vi "Save File Create Default DOE Setup File.vi"(11 "Config Path":path=path "C:/GE/Washer DOE/WasherDOEConfig.csv") -> ()   [LabVIEW 2016, in "File Setup.lvlib"]
uses:
  File Setup.lvlib
  <vilib>/Utility/file.llb/Read From Spreadsheet File (string).vi
  <vilib>/Utility/file.llb/Write To Spreadsheet File (string).vi
panel:
  out "INI File Exists":bool
  out "CSV File Exists":bool
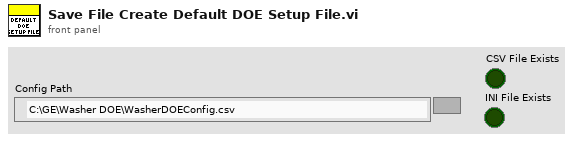
[diagram p1: front panel]
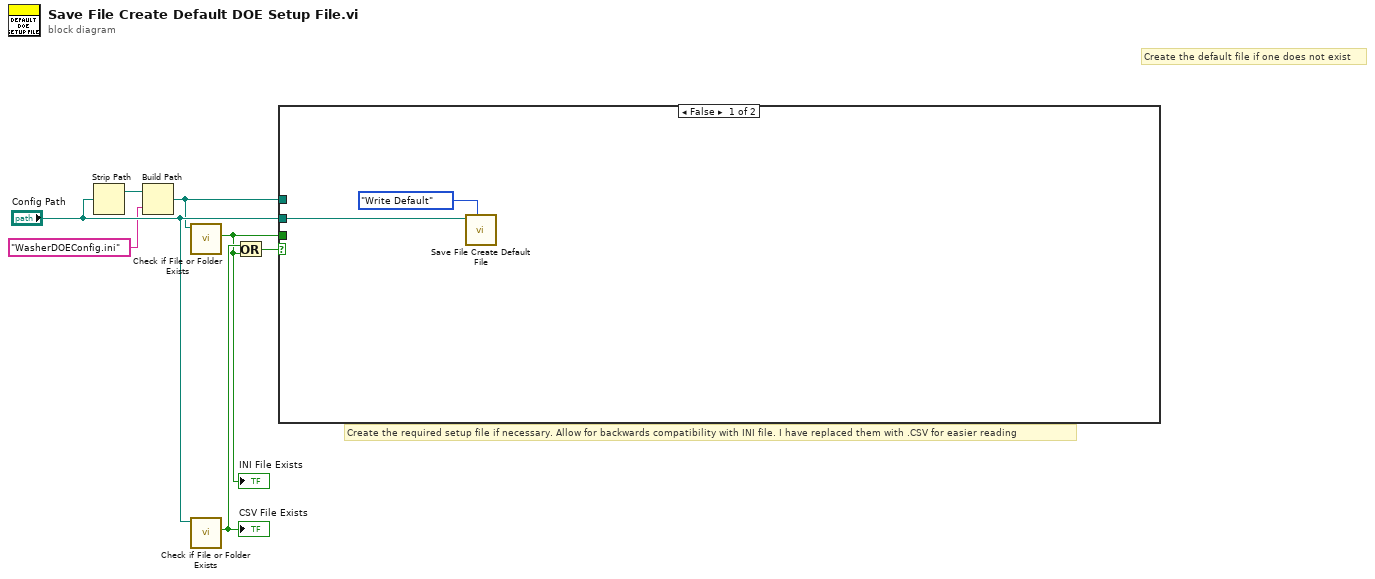
[diagram p0: block diagram]
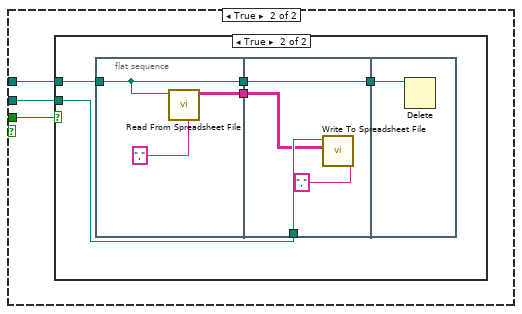
[diagram p2: hidden frame]
diagram:
  # "Create the required setup file if necessary. Allow for backwards compatibility with INI file. I have replaced them with .CSV for easier reading"
  # "Create the default file if one does not exist"
  n1 = Strip Path(path="Config Path") -> (stripped path=w4:path)  [unwired: 1 out]
  n2 = Build Path(base path=w4, name or relative path="WasherDOEConfig.ini") -> (appended path=w2:path)
  n3 = call <vilib>:"Check if File or Folder Exists.vi"("path"=w2) -> ("file or folder exists?"=w1:bool)  [unwired: 8 in, 2 out]
  "INI File Exists" <- w1
  n4 = call <vilib>:"Check if File or Folder Exists.vi"("path"="Config Path") -> ("file or folder exists?"=w7:bool)  [unwired: 8 in, 2 out]
  "CSV File Exists" <- w7
  n5 = Or(x=w7, y=w1) -> (x .or. y?=w6:bool)
  n6 = case shown="False" w6 {
    tunnel: "Config Path" -> [w9 w10]
    tunnel: w2 -> [_ w12]
    tunnel: w1 -> [_ w11]
    frame False {
      n7 = call "Save File Create Default File.vi"("Type"=enum16{"Pass Default", "Write Default"}."Write Default", "Config Path"=w9) -> ()  [unwired: 9 in, 1 out]
    }
    frame True {
      n8 = case shown="True" w11 {
        tunnel: w12 -> [_ w17]
        tunnel: w10 -> [_ w15]
        frame False {
        }
        frame True {
          n9 = flat-sequence {
            tunnel: w17 -> [w18]
            tunnel: [w20] -> w16
            tunnel: [w18] -> w14
            tunnel: w16 -> [w22]
            tunnel: w15 -> [w24]
            tunnel: w14 -> [w21]
            tunnel: [w21] -> w13
            tunnel: w13 -> [w25]
            frame #0 {
              n10 = call-poly <vilib>:"Read From Spreadsheet File.vi"("delimiter (\\t)"="," ("delimiter (\\t)"), "file path (dialog if empty)"=w18) -> ("all rows"=w20:string[][])  [unwired: 5 in, 4 out]
            }
            frame #1 {
              n11 = call-poly <vilib>:"Write To Spreadsheet File.vi"("delimiter (\\t)"="," ("delimiter (\\t)"), "2D data"=w22, "file path (dialog if empty)"=w24) -> ()  [unwired: 5 in, 1 out]
            }
            frame #2 {
              n12 = Delete(path (use dialog)=w25) -> ()  [unwired: 4 in, 3 out]
            }
          }
        }
      }
    }
  }
